vi "InsertionLoss.vi"() -> ()   [LabVIEW 2022 SP3]
uses:
  ScanningControl/Digitizers/-DigitizerRoutines/Digitizer.ctl
  Instance           6 21Saved   InsertionLoss .vi
  <vilib>/Utility/file.llb/Write To Spreadsheet File (DBL).vi
panel:
  in  "Main Digitizer":T1=enum."NI Digitizer"
  in  "Tabor (V)":dbl=0.05 format="%#.2f"
  out "RCV raw":dbl[](array[numeric]) format="%.2f"
  out "none + pk and -pk":dbl[][](graph)
  in  "Boolean":bool=TRUE
  out "none pk-pk":cluster{dbl[], dbl[]}(graph)
  in  "Tab Control":enum32{"Rcv", "Xmit"}(tab)
  in  "Corrections Rcv(dB)":dbl format="%.2f"
  in  "RT water path mm":dbl format="%.2f"
  in  "Corrections (dB)":dbl format="%.2f"
  out "ILoss":cluster{dbl[], dbl[]}(graph)
  out "Xmit":cluster{dbl[], dbl[]}(graph)
  in  "Save":bool
  out "RF data Out":T2={"Sampling Rate"=0, "Delay (micro s)"=0.5, "rf points per line"=500} {"Delay (micro s)" format="%.2f"}
  out "Rcv":cluster{dbl[], dbl[]}(graph)
  in  "Freq Step MHz":dbl=1.0 format="%.2f"
  in  "Steps":i32=60
  in  "Start frequency (MHz)":dbl=10.0 format="%.2f"
  # "-32.5 dB normally used for receive"
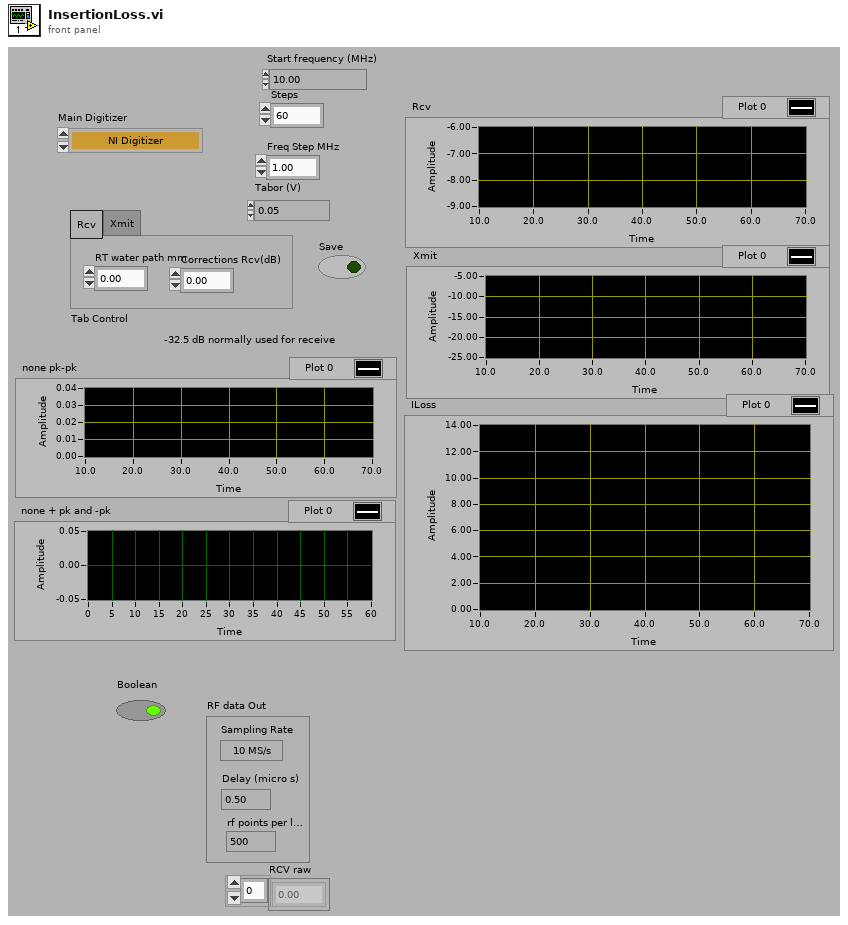
[diagram p1: front panel]
types:
  T1 = typedef "Digitizer.ctl" = enum16{"Acqiris Digitizer", "NI Digitizer", "LeCroy", "GaGe", "AlazarTech", "No Digitizer", "Teledyne"}
  T2 = cluster{"Sampling Rate":u16, "Delay (micro s)":dbl, "rf points per line":u16}
  T3 = cluster{"Voltage Full Scale (pp)":u16, i32, "Coupling 2":u16}
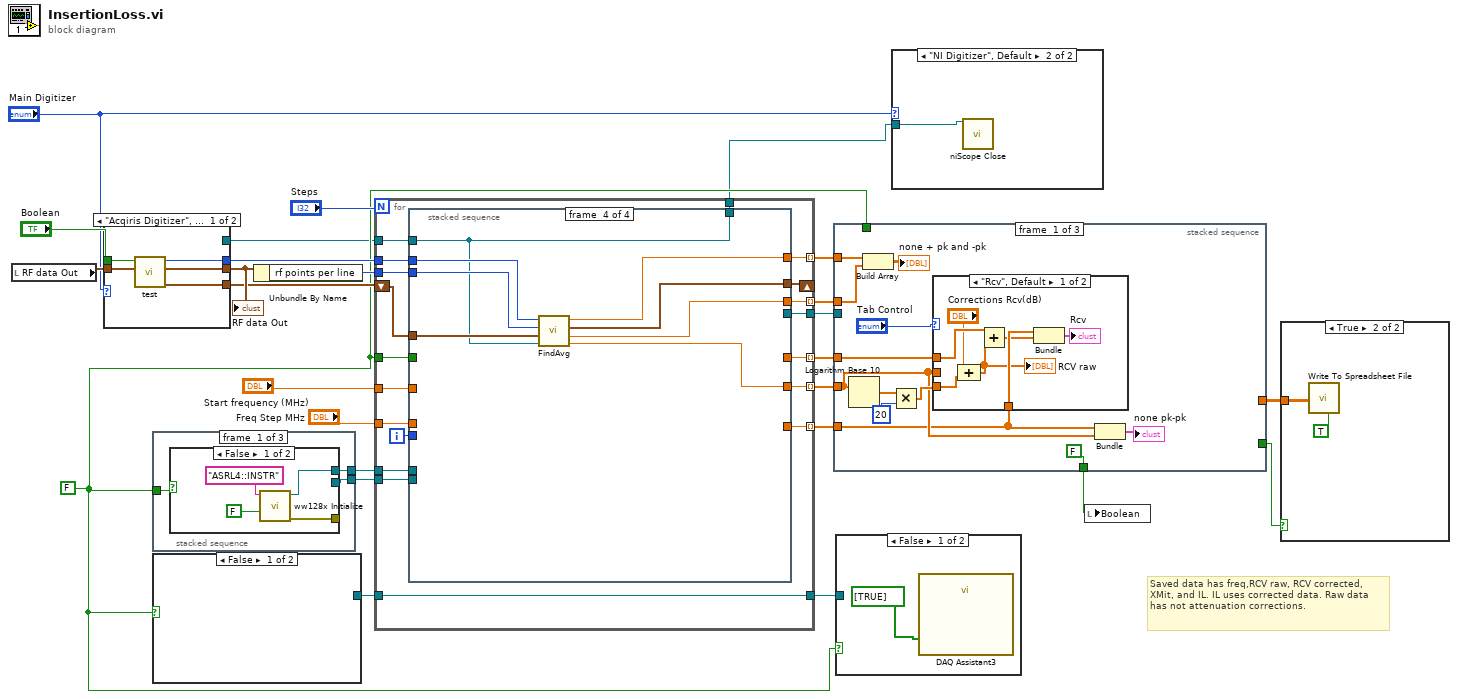
[diagram p0: block diagram]
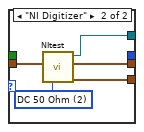
[diagram p3: hidden frame]
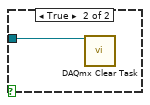
[diagram p4: hidden frame]
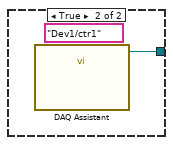
[diagram p5: hidden frame]
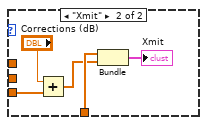
[diagram p6: hidden frame]
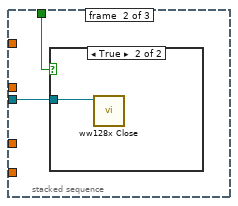
[diagram p7: hidden frame]
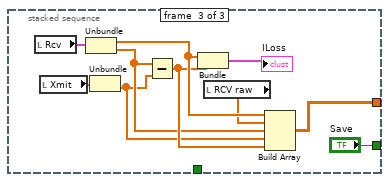
[diagram p9: hidden frame]
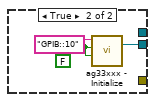
[diagram p11: hidden frame]
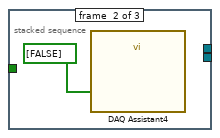
[diagram p12: hidden frame]
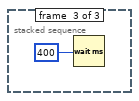
[diagram p13: hidden frame]
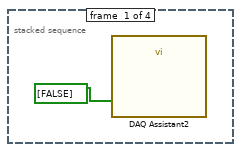
[diagram p14: hidden frame]
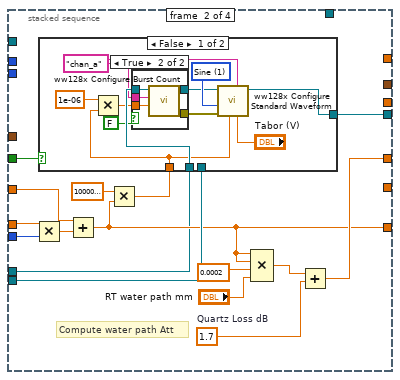
[diagram p15: hidden frame]
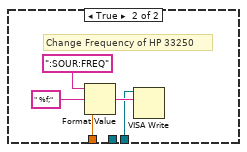
[diagram p17: hidden frame]
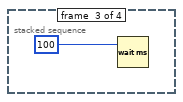
[diagram p18: hidden frame]
diagram:
  w4 = FALSE
  # "Saved data has freq,RCV raw, RCV corrected, XMit, and IL. IL uses corrected data. Raw data has not attenuation corrections."
  n1 = local read "RF data Out"() -> (w21:T2)
  n2 = case shown="\"Acqiris Digitizer\", Default" "Main Digitizer" {
    tunnel: [w31 _] -> w22
    tunnel: w21 -> [w30 w34]
    tunnel: "Boolean" -> [w29 _]
    tunnel: [w28 w35] -> w12
    tunnel: [w27 w36] -> w11
    tunnel: [_ w32] -> w3
    frame "Acqiris Digitizer", Default {
      n3 = call "test.vi"("RF data Sampling"=w30, "Boolean"=w29) -> ("voltage range"=w27:T3, "RF data Out"=w28:T2, "ID"=w31:i32)  [unwired: 1 in, 2 out]
    }
    frame "NI Digitizer" {
      w33 = u16 2 items=["DC 1 MOhm", "AC 1 MOhm", "DC 50 Ohm", "AC 50 OHM"] ("Coupling")
      n4 = call "NItest.vi"("Coupling"=w33, "RF data Sampling"=w34) -> ("voltage range"=w36:T3, "RF data Out"=w35:T2, "ID"=w32:refnum<k15>)  [unwired: 1 in, 2 out]
    }
  }
  "RF data Out" <- w12
  n5 = stacked-sequence {
    tunnel: [w39 _ _] -> w26
    tunnel: w4 -> [w38 _ _]
    tunnel: [w37 _ _] -> w6
    frame #0 {
      n6 = case shown="False" w38 {
        tunnel: [_ w45] -> w39
        tunnel: [w42 _] -> w37
        tunnel: [w40 _] -> _
        frame False {
          n7 = call <instrlib>:"ww128x Initialize.vi"("reset device (Yes)"=FALSE ("reset device"), "resource name"="ASRL4::INSTR") -> ("error out"=w40:errorcluster, "instrument handle out"=w42:refnum<k15>)  [unwired: 2 in, 6 out]
        }
        frame True {
          w44 = FALSE
          n8 = call <instrlib>:"ag33xxx - Initialize.vi"("Reset (T: Reset)"=w44, "ID Query (T: Check)"=w44, "Instrument Resource Name"="GPIB::10") -> ("dup VISA session"=w45:refnum<visa-resource-name>)  [unwired: 1 in, 7 out]
        }
      }
    }
    frame #1 {
      n9 = call "DAQ Assistant4"("data"=bool[] [FALSE]) -> ()  [unwired: 3 in, 16 out]
    }
    frame #2 {
      n10 = Wait (ms)(milliseconds to wait=400) -> ()  [unwired: 1 out]
    }
  }
  n11 = case shown="False" w4 {
    tunnel: [_ w49] -> w7
    frame False {
    }
    frame True {
      (unwired) tag "Dev1/ctr1" ("counter")
      n12 = call "DAQ Assistant"() -> ("task out"=w49:refnum<k21>)  [unwired: 2 in, 17 out]
    }
  }
  n13 = Unbundle By Name(w12) -> ("rf points per line"=w17:u16)
  n14 = for {
    N: "Steps" -> [_]
    tunnel: w26 -> [w68]
    tunnel: "Freq Step MHz" -> [w66]
    tunnel: "Start frequency (MHz)" -> [w65]
    tunnel: [w64] -> w19 mode=indexing
    tunnel: [w63] -> w23 mode=indexing
    tunnel: w22 -> [w62]
    tunnel: [w61] -> w20 mode=indexing
    tunnel: w17 -> [w60]
    tunnel: [w59] -> w14 mode=indexing
    tunnel: [w58] -> w13 mode=indexing
    shift-right: [w56] -> _
    shift-left: w11 -> [w57]
    tunnel: [w55] -> w8
    tunnel: w7 -> [w55]
    tunnel: w4 -> [w54]
    tunnel: w6 -> [w53]
    tunnel: [w52] -> w5
    tunnel: w3 -> [w50]
    tunnel: [w51] -> w2
    i -> [w67]
    n15 = stacked-sequence {
      tunnel: w68 -> [_ w85 _ _]
      tunnel: w67 -> [_ w84 _ _]
      tunnel: w66 -> [_ w83 _ _]
      tunnel: w65 -> [_ w81 _ _]
      tunnel: [_ _ _ w110] -> w64
      tunnel: [_ w74 _ _] -> w63
      tunnel: w62 -> [_ _ _ w116]
      tunnel: [_ w76 _ _] -> w61
      tunnel: w60 -> [_ _ _ w115]
      tunnel: [_ _ _ w114] -> w59
      tunnel: [_ _ _ w113] -> w58
      tunnel: w57 -> [_ _ _ w112]
      tunnel: [_ _ _ w111] -> w56
      tunnel: w54 -> [_ w72 _ _]
      tunnel: w53 -> [_ w71 _ _]
      tunnel: [_ w70 _ _] -> w52
      tunnel: w50 -> [_ _ _ w109]
      tunnel: [_ _ _ w109] -> w51
      frame #0 {
        n16 = call "DAQ Assistant2"("data"=bool[] [FALSE]) -> ()  [unwired: 3 in, 16 out]
      }
      frame #1 {
        w77 = 1.7  # Quartz Loss dB
        # "Compute water path Att"
        n17 = Multiply(x=w83, y=w84) -> (x*y=w82:dbl)
        n18 = Add(x=w81, y=w82) -> (x+y=w74:dbl)
        n19 = Multiply(x=1000000.0, y=w74) -> (x*y=w73:dbl)
        n20 = case shown="False" w72 {
          tunnel: w85 -> [_ w103]
          tunnel: w73 -> [w89 w104]
          tunnel: w71 -> [w93 _]
          tunnel: [w91 _] -> w70
          frame False {
            w86 = "chan_a" ("channel name (\"CHAN_A\")")
            w96 = 1 items=["Sine"=1, "Square"=2, "Triangle"=3, "Ramp Up"=4, "Ramp Down"=5, "DC"=6, "Ramp"=1001, "Pulse"=1005, "Sync"=1002, "Gaussian"=1003, "Exponential"=1004, "Noise"=1006] ("waveform")
            n21 = Multiply(x=1e-06, y=w89) -> (x*y=w88:dbl)
            n22 = case shown="True" FALSE {
              tunnel: [w97 w102] -> w95
              tunnel: [_ w101] -> w94
              tunnel: w93 -> [w97 w100]
              tunnel: w88 -> [_ w99]
              tunnel: w86 -> [_ w98]
              frame False {
              }
              frame True {
                n23 = call <instrlib>:"ww128x Configure Burst Count.vi"("burst count (2)"=w99, "channel name (\"CHAN_A\")"=w98, "instrument handle"=w100) -> ("error out"=w101:errorcluster, "instrument handle out"=w102:refnum<k15>)  [unwired: 1 in, 6 out]
              }
            }
            n24 = call <instrlib>:"ww128x Configure Standard Waveform.vi"("amplitude"="Tabor (V)", "frequency"=w89, "error in (no error)"=w94, "waveform"=w96, "channel name"=w86, "instrument handle"=w95) -> ("instrument handle out"=w91:refnum<k15>)  [unwired: 2 in, 3 out]
          }
          frame True {
            # "Change Frequency of HP 33250"
            n25 = Format Value(string ("")=":SOUR:FREQ", format string=" %f;", value (0)=w104) -> (output string=w105:string)
            n26 = VISA Write(VISA resource name=w103, write buffer=w105) -> ()  [unwired: 1 in, 3 out]
          }
        }
        n27 = Compound Arithmetic op=MULTIPLY(w74, w74, 0.0002, "RT water path mm") -> (w78:dbl)
        n28 = Add(x=w78, y=w77) -> (x+y=w76:dbl)
      }
      frame #2 {
        n29 = Wait (ms)(milliseconds to wait=100) -> ()  [unwired: 1 out]
      }
      frame #3 {
        n30 = call "FindAvg.vi"("ID"=w109, "voltage range in"=w112, "rf points per line"=w115, "Acqiris ID"=w116) -> ("Vpp"=w110:dbl, "Vmin"=w113:dbl, "voltage range out"=w111:T3, "Vmax"=w114:dbl)  [unwired: 1 in]
      }
    }
  }
  n31 = stacked-sequence {
    tunnel: w23 -> [w120 _ _]
    tunnel: w20 -> [w128 _ _]
    tunnel: w19 -> [w121 _ _]
    tunnel: [_ _ w149] -> w18
    tunnel: [FALSE _ _] -> w15
    tunnel: w14 -> [w118 _ _]
    tunnel: w13 -> [w117 _ _]
    tunnel: [_ _ "Save"] -> w9
    tunnel: w5 -> [_ w142 _]
    tunnel: w4 -> [_ w141 _]
    frame #0 {
      n32 = Logarithm Base 10(1:w121) -> (0:w127:dbl[])
      n33 = Build Array(w118, w117) -> (→"none + pk and -pk":dbl[][])
      n34 = Multiply(x=w127, y=20) -> (x*y=w125:dbl[])
      n35 = case shown="\"Rcv\", Default" "Tab Control" {
        tunnel: w125 -> [w130 w138]
        tunnel: w128 -> [w133 _]
        tunnel: w120 -> [w134 w137]
        tunnel: w121 -> [_ _]
        frame "Rcv", Default {
          n36 = Compound Arithmetic op=ADD("Corrections Rcv(dB)", w130) -> (w129:dbl[])
          "RCV raw" <- w129
          n37 = Add(x=w133, y=w129) -> (x+y=w132:dbl[])
          n38 = Bundle(w134, w132) -> (→"Rcv":cluster{dbl[], dbl[]})  [unwired: 1 out]
        }
        frame "Xmit" {
          n39 = Add(x="Corrections (dB)", y=w138) -> (x+y=w136:dbl[])
          n40 = Bundle(w137, w136) -> (→"Xmit":cluster{dbl[], dbl[]})  [unwired: 1 out]
        }
      }
      n41 = Bundle(w120, w121) -> (→"none pk-pk":cluster{dbl[], dbl[]})  [unwired: 1 out]
    }
    frame #1 {
      n42 = case shown="True" w141 {
        tunnel: w142 -> [_ w143]
        frame False {
        }
        frame True {
          n43 = call <instrlib>:"ww128x Close.vi"("instrument handle"=w143) -> ()  [unwired: 1 in, 10 out]
        }
      }
    }
    frame #2 {
      n44 = local read "Rcv"() -> (w152:cluster{dbl[], dbl[]})
      n45 = local read "Xmit"() -> (w151:cluster{dbl[], dbl[]})
      n46 = Unbundle(w152) -> (w150:dbl[], w146:dbl[])
      n47 = Unbundle(w151) -> (w145:dbl[])  [unwired: 1 out]
      n48 = Subtract(x=w146, y=w145) -> (x-y=w148:dbl[])
      n49 = Bundle(w150, w148) -> (→"ILoss":cluster{dbl[], dbl[]})  [unwired: 1 out]
      n50 = local read "RCV raw"() -> (w147:dbl[])
      n51 = Build Array(w150, w147, w146, w145, w148) -> (w149:dbl[][])
    }
  }
  n52 = case shown="False" w4 {
    tunnel: w8 -> [_ w155]
    frame False {
      n53 = call "DAQ Assistant3"("data"=bool[] [TRUE]) -> ()  [unwired: 3 in, 16 out]
    }
    frame True {
      n54 = call <vilib>:"DAQmx Clear Task.vi"("task in"=w155) -> ()  [unwired: 1 in, 14 out]
    }
  }
  n55 = case shown="\"NI Digitizer\", Default" "Main Digitizer" {
    tunnel: w2 -> [_ w156]
    frame "Acqiris Digitizer" {
    }
    frame "NI Digitizer", Default {
      n56 = call <instrlib>:"niScope Close.vi"("instrument handle"=w156) -> ()  [unwired: 1 in, 14 out]
    }
  }
  n57 = local write "Boolean"(w15) -> ()
  n58 = case shown="True" w9 {
    tunnel: w18 -> [_ w157]
    frame False {
    }
    frame True {
      n59 = call-poly <vilib>:"Write To Spreadsheet File.vi"("transpose? (no:F)"=TRUE, "2D data"=w157) -> ()  [unwired: 4 in, 3 out]
    }
  }
